vi "Toggle on Press.vi"(11 "Boolean":bool) -> (3 "toggle on press":bool)   [LabVIEW 2018]
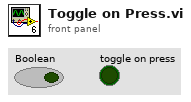
[diagram p1: front panel]
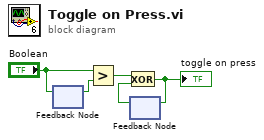
[diagram p0: block diagram]
diagram:
  n1 = feedback #1() -> (w1:bool)  [unwired: 1 in]
  n2 = feedback-in #1("Boolean") -> ()
  n3 = Greater?(x="Boolean", y=w1) -> (0:w3:bool)
  n4 = feedback #2() -> (w4:bool)  [unwired: 1 in]
  n5 = Exclusive Or(1:w4, 2:w3) -> (0:w2:bool)
  "toggle on press" <- w2
  n6 = feedback-in #2(w2) -> ()
